vi "Assinante.vi"() -> ()   [LabVIEW 2018]
uses:
  RxTx/RxTx.lvclass
panel:
  out "error out":errorcluster
  in  "Queue RX":refnum<class "RxTx.lvclass">
  out "Received Publication":string
  in  "stop":bool
  # "SUB endpoint"
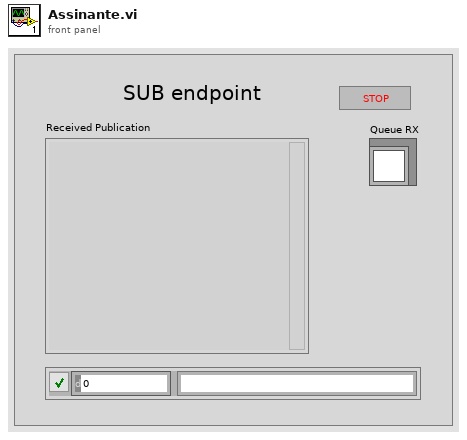
[diagram p1: front panel]
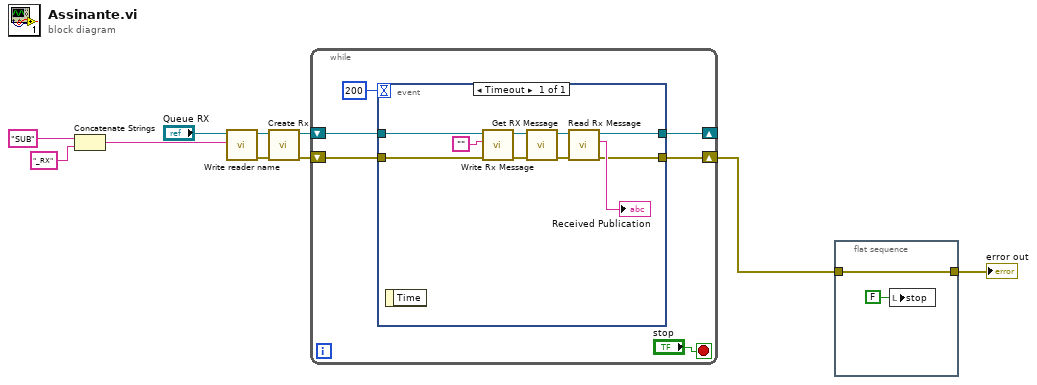
[diagram p0: block diagram]
diagram:
  n1 = Concatenate Strings("SUB" ("string"), "_RX" ("string")) -> (w4:string)
  n2 = call-dynamic "Write reader name.vi"("RX name"=w4, "RxTx in"="Queue RX") -> ("error out"=w7:errorcluster, "RxTx out"=w8:refnum<class "RxTx.lvclass">)  [unwired: 8 in]
  n3 = call "Create Rx.vi"("error in (no error)"=w7, "RxTx in"=w8) -> ("error out"=w6:errorcluster, "RxTx out"=w9:refnum<class "RxTx.lvclass">)  [unwired: 8 in]
  n4 = while {
    shift-right: [w13] -> _
    shift-left: w9 -> [w14]
    shift-right: [w11] -> w1
    shift-left: w6 -> [w12]
    stop <- "stop" stop-if-true
    n5 = event shown="[0] Timeout" {
      selector: _ -> [_]
      dyn-events: _ -> [_]
      timeout: 200 -> [_]
      tunnel: w14 -> [w23]
      tunnel: [w21] -> w13
      tunnel: w12 -> [w18]
      tunnel: [w17] -> w11
      event Timeout {
        n6 = event-data() -> ()  [unwired: 1 in, 1 out]
        n7 = call "Write Rx Message.vi"("error in (no error)"=w18, "Rx Message"="", "RxTx in"=w23) -> ("error out"=w20:errorcluster, "RxTx out"=w22:refnum<class "RxTx.lvclass">)  [unwired: 7 in]
        n8 = call "Get RX Message.vi"("error in (no error)"=w20, "RxTx in"=w22) -> ("error out"=w24:errorcluster, "RxTx out"=w26:refnum<class "RxTx.lvclass">)  [unwired: 7 in, 1 out]
        n9 = call "Read Rx Message.vi"("error in (no error)"=w24, "RxTx in"=w26) -> ("error out"=w17:errorcluster, "Rx Message"=→"Received Publication":string, "RxTx out"=w21:refnum<class "RxTx.lvclass">)  [unwired: 7 in]
      }
    }
  }
  n10 = flat-sequence {
    tunnel: w1 -> [w28]
    tunnel: [w28] -> w5
    frame #0 {
      n11 = local write "stop"(FALSE ("stop")) -> ()
    }
  }
  "error out" <- w5
